vi "initializeSharedVars.vi"(8 "error in (no error)":errorcluster, 11 "FakePressureController in":refnum<class "TDK-Lambda Z Bipolar.lvclass">) -> (0 "error out":errorcluster, 3 "FakePressureController out":refnum<class "TDK-Lambda Z Bipolar.lvclass">)   [LabVIEW 2020, in "TDK-Lambda Z Bipolar.lvclass"]
uses:
  TDK-Lambda Z Bipolar.lvclass
  TDK-Lambda Z Bipolar.lvclass/TDK-Lambda Z Bipolar.ctl
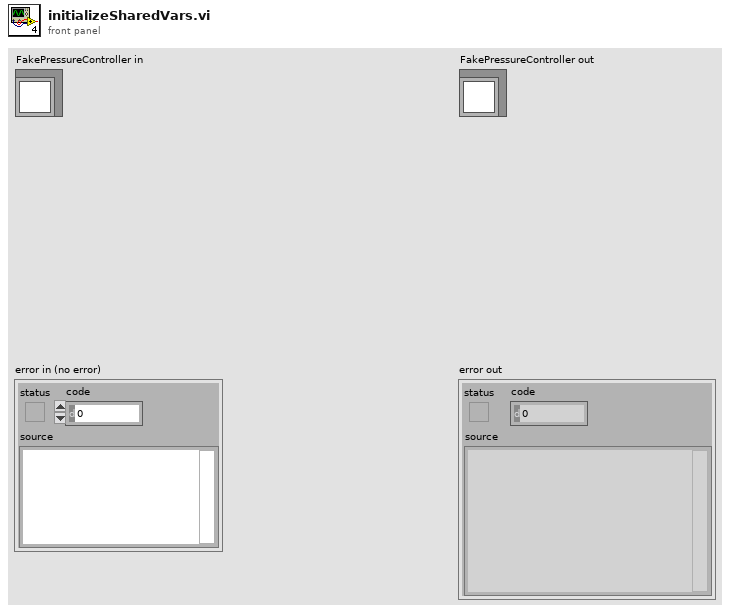
[diagram p1: front panel]
types:
  T1 = cluster{"Read Access":enum8{"Allowed", "Required", "None"}, "Write Access":enum8{"Allowed", "Required", "None"}}
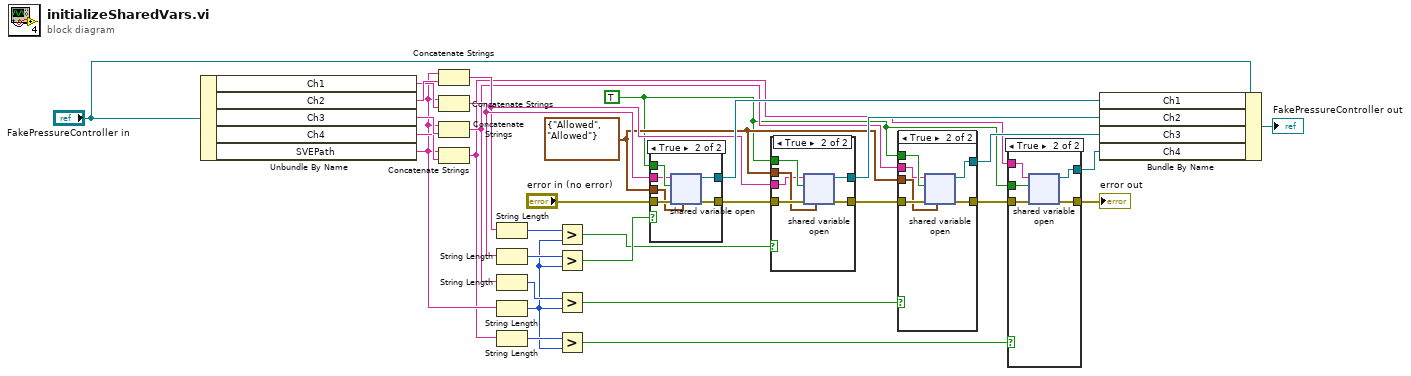
[diagram p0: block diagram]
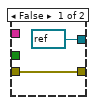
[diagram p2: hidden frame]
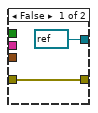
[diagram p3: hidden frame]
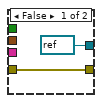
[diagram p4: hidden frame]
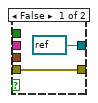
[diagram p5: hidden frame]
diagram:
  w10 = T1 {"Read Access"=enum."Allowed", "Write Access"=enum."Allowed"} ("access")
  w4 = TRUE
  n1 = Unbundle By Name("FakePressureController in") -> ("Ch1"=w23:string, "Ch2"=w31:string, "Ch3"=w30:string, "Ch4"=w29:string, "SVEPath"=w18:string)
  n2 = Concatenate Strings(w18, w31) -> (w16:string)
  n3 = Concatenate Strings(w18, w23) -> (w19:string)
  n4 = Concatenate Strings(w18, w30) -> (w13:string)
  n5 = Concatenate Strings(w18, w29) -> (w3:string)
  n6 = String Length(string=w16) -> (length=w20:i32)
  n7 = String Length(string=w19) -> (length=w24:i32)
  n8 = String Length(string=w13) -> (length=w14:i32)
  n9 = String Length(string=w18) -> (length=w6:i32)
  n10 = String Length(string=w3) -> (length=w8:i32)
  n11 = Greater?(x=w20, y=w6) -> (0:w17:bool)
  n12 = Greater?(x=w24, y=w6) -> (0:w22:bool)
  n13 = Greater?(x=w14, y=w6) -> (0:w12:bool)
  n14 = Greater?(x=w8, y=w6) -> (0:w7:bool)
  n15 = case shown="True" w22 {
    tunnel: w4 -> [_ w39]
    tunnel: "error in (no error)" -> [w33 w38]
    tunnel: w10 -> [_ w37]
    tunnel: w19 -> [_ w36]
    tunnel: [refnum<k21> refnum w35] -> w25
    tunnel: [w33 w34] -> w21
    frame False {
    }
    frame True {
      n16 = shared-variable-open(w36, w38, w39, w37) -> (w35:refnum<k21>, w34:errorcluster)
    }
  }
  n17 = case shown="True" w17 {
    tunnel: w4 -> [_ w47]
    tunnel: w21 -> [w41 w46]
    tunnel: w10 -> [_ w45]
    tunnel: w16 -> [_ w44]
    tunnel: [refnum<k21> refnum w43] -> w15
    tunnel: [w41 w42] -> w11
    frame False {
    }
    frame True {
      n18 = shared-variable-open(w44, w46, w47, w45) -> (w43:refnum<k21>, w42:errorcluster)
    }
  }
  n19 = case shown="True" w12 {
    tunnel: w4 -> [_ w55]
    tunnel: w11 -> [w49 w54]
    tunnel: w10 -> [_ w53]
    tunnel: w13 -> [_ w52]
    tunnel: [refnum<k21> refnum w51] -> w9
    tunnel: [w49 w50] -> w5
    frame False {
    }
    frame True {
      n20 = shared-variable-open(w52, w54, w55, w53) -> (w51:refnum<k21>, w50:errorcluster)
    }
  }
  n21 = case shown="True" w7 {
    tunnel: [refnum<k21> refnum w62] -> w2
    tunnel: [w56 w61] -> w1
    tunnel: w5 -> [w56 w60]
    tunnel: w4 -> [_ w59]
    tunnel: w3 -> [_ w58]
    frame False {
    }
    frame True {
      n22 = shared-variable-open(w58, w60, w59) -> (w62:refnum<k21>, w61:errorcluster)  [unwired: 1 in]
    }
  }
  "error out" <- w1
  n23 = Bundle By Name(cluster="FakePressureController in", "Ch1"=w25, "Ch2"=w15, "Ch3"=w9, "Ch4"=w2) -> (→"FakePressureController out":refnum<class "TDK-Lambda Z Bipolar.lvclass">)
